vi "calculation.vi"(0 "power":dbl[](array[numeric]), 2 "voltage":dbl[](array[numeric]), 4 "|current|":dbl[](array[numeric]), 6 "current":dbl[](array[numeric]), 11 "|voltage|":dbl[](array[numeric]), 15 "Device Area (cm^2)":dbl, 19 "Light  Intensity (mW/cm^2)":dbl) -> (10 "Jsc":dbl, 14 "Isc":dbl, 20 "IVmax":dbl, 22 "FF":dbl, 24 "Pce":dbl, 26 "Voc":dbl)   [LabVIEW 2014]
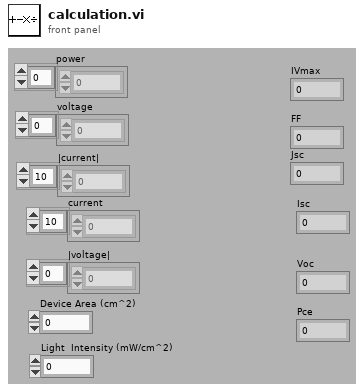
[diagram p1: front panel]
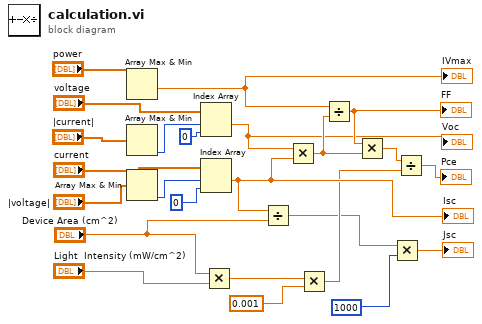
[diagram p0: block diagram]
diagram:
  n1 = Array Max & Min(array="power") -> (min value=w10:dbl)  [unwired: 3 out]
  "IVmax" <- w10
  n2 = Array Max & Min(array="|current|") -> (min index (indices)=w17:i32)  [unwired: 3 out]
  n3 = Array Max & Min(array="|voltage|") -> (min index (indices)=w18:i32)  [unwired: 3 out]
  n4 = Index Array(array="voltage", index #1=w17, index #2=0 ("index")) -> (element #1=w21:dbl)  [unwired: 1 out]
  "Voc" <- w21
  n5 = Index Array(array="current", index #1=w18, index #2=0 ("index")) -> (element #1=w9:dbl)  [unwired: 1 out]
  "Isc" <- w9
  n6 = Multiply(x="Device Area (cm^2)", y="Light  Intensity (mW/cm^2)") -> (x*y=w6:dbl)
  n7 = Divide(x=w9, y="Device Area (cm^2)") -> (x/y=w2:dbl)
  n8 = Multiply(x=w21, y=w9) -> (x*y=w23:dbl)
  n9 = Multiply(x=w6, y=0.001) -> (x*y=w4:dbl)
  n10 = Divide(x=w10, y=w23) -> (x/y=w22:dbl)
  "FF" <- w22
  n11 = Multiply(x=w22, y=w23) -> (x*y=w24:dbl)
  n12 = Multiply(x=w2, y=1000) -> (x*y=→"Jsc":dbl)
  n13 = Divide(x=w24, y=w4) -> (x/y=→"Pce":dbl)
